vi "Mock MVA VI.vi"(9 "Datum Value":variant, 10 "Datum Name":string) -> ()   [LabVIEW 2019]
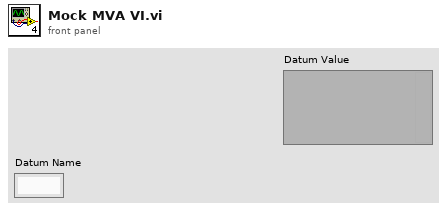
[diagram p1: front panel]
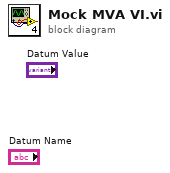
[diagram p0: block diagram]
diagram:
